vi "Calibrate Probe Tube.vi"(5 "Right":string="SN24", 7 "Left":string="SN31", 9 "Outputs":T14[](array[typedef])=[{"Name"="Right primary", "Device"="Dev1/ao0"}, {"Name"="Right secondary", "Device"="Dev1/ao1"}, {"Name"="Left primary", "Device"=""}, {"Name"="Left secondary", "Device"=""}, {"Name"="Shaker", "Device"=""}, {"Name"="Background", "Device"=""}], 11 "Inputs":T14[](array[typedef])=[{"Name"="Probe Mic Right", "Device"="Dev1/ai0"}, {"Name"="Probe Mic Left", "Device"=""}, {"Name"="Cal Mic", "Device"="Dev1/ai1"}, {"Name"="ABR", "Device"=""}, {"Name"="CAP Right", "Device"=""}, {"Name"="CAP Left", "Device"=""}, {"Name"="Accelerometer", "Device"=""}, {"Name"="Temperature", "Device"=""}, {"Name"="Heart rate", "Device"=""}]) -> ()   [LabVIEW 2020]
uses:
  <vilib>/printing/EasyPrintingControls.llb/layout_options.ctl
  <vilib>/printing/EasyPrintingControls.llb/orientation.ctl
  <vilib>/printing/EasyPrintingControls.llb/panel_scaling_for_page.ctl
  <vilib>/printing/EasyPrintingControls.llb/margins.ctl
  <vilib>/printing/EasyPrintingControls.llb/margin_values.ctl
  <vilib>/printing/EasyPrintingControls.llb/measurement_system.ctl
  <vilib>/printing/EasyPrintingControls.llb/printer_options.ctl
  <vilib>/printing/EasyPrintingControls.llb/printing_method.ctl
  <vilib>/printing/EasyPrintingControls.llb/color_or_monochrome.ctl
  <vilib>/printing/EasyPrintingControls.llb/page_header_options.ctl
  <vilib>/printing/EasyPrintingControls.llb/page_headers.ctl
  <vilib>/printing/EasyPrintingControls.llb/page_header_content_options.ctl
  epl-vi-lib/Utility VIs/Controls/KLegend/KLegend.xctl
  Common VIs/Typedefs/CAL-Endpoint.ctl
  Typedefs/PTC-Parameters.ctl
  Common VIs/Typedefs/CAL-Stimulus.ctl
  Typedefs/PTC-Queue Data.ctl
  Typedefs/PTC-Response.ctl
  epl-vi-lib/PXI DAQ VIs/AIDI/Typedefs/AIDI-Action.ctl
  <vilib>/printing/EasyPrintingControls.llb/contents.ctl
  7e04b9d2-1ebf-4042-b86f-09db3b0598e0.vi
  3dd90dd6-0296-4ee9-b2b6-3c947d5e5bcc.vi
  Common VIs/Typedefs/CAL-Globals.vi
  epl-vi-lib/Utility VIs/Math VIs/FFT x(t) to dB,Degrees (2D).vi
  epl-vi-lib/Utility VIs/Conversion VIs/Create Waveform Cluster (2D).vi
  epl-vi-lib/Utility VIs/File IO VIs/FileIO-Create Backup.vi
  epl-vi-lib/Utility VIs/File IO VIs/Append to Text File.vi
  <vilib>/printing/EasyPrinting.llb/Easy Print VI Panel or Documentation (refnum).vi
  <vilib>/Utility/NIReport.llb/NI_ReportGenerationCore.lvlib
panel:
  out "Acquired":i32=256
  in  "layout options":T1={"orientation (unchanged)"=0, "panel scaling for page (unchanged)"=0, "margins"={"override VI margins (false)"=FALSE, "margins (1.00)"={"top"=1.0, "left"=1.0, "right"=1.0, "bottom"=1.0}, "measurement system (default)"=0}, "printer options"={"destination printer name (current)"="", "printing method (unchanged)"=0, "color or monochrome (unchanged)"=0}, "page header options"={"page headers (unchanged)"=0, "page header content options"={"Include VI Name"=TRUE, "Include VI Path"=TRUE, "Include Last Modification Date"=TRUE, "Include Date Printed"=TRUE, "Include Page Number"=TRUE, "Include VI Icon"=TRUE}}} {"page header options"."page headers (unchanged)" items=["Unchanged", "Include page headers", "Do not include page headers"]; "printer options"."color or monochrome (unchanged)" items=["Unchanged", "Color/grayscale", "Monochrome"]; "printer options"."printing method (unchanged)" items=["Unchanged", "Standard", "PostScript", "Bitmap"]; "panel scaling for page (unchanged)" items=["Unchanged", "No Scaling", "Scale front panel to fit"]; "orientation (unchanged)" items=["Unchanged", "portrait", "landscape"]; "margins"."measurement system (default)" items=["Default", "US", "Metric"]; "margins"."margins (1.00)"."right" format="%.2f"; "margins"."margins (1.00)"."bottom" format="%.2f"; "margins"."margins (1.00)"."top" format="%.2f"; "margins"."margins (1.00)"."left" format="%.2f"}
  in  "Correction curve":path
  in  "Measure":bool
  out "(mV/Pa)":dbl=40.0 format="%#_4g"
  in  "Acoustic System ID":string="SN31"
  in  "Ear":enum16{"Right", "Left"}(ring)
  in  "Probe Mic Gain (dB)":dbl
  in  "Cal Mic Gain (dB)":dbl=40.0
  in  "Stimulus":T13={"Freq Step (Hz)"=50.0, "Stimulus"=enum."Chirp", "Attenuation (dB)"=30.0, "Sample Rate (Hz)"=100000.0}
  in  "Averages":i32=256
  in  "Cal Mic Sens":dbl=-146.12351367888365 caption="(dB V/SPL)" format="%.2f"
  in  "RETURN":bool
  in  "START":bool
  in  "STOP":bool
  out "result":cluster{"Path":path, "error":errorcluster}
  in  "Data tabs":enum32{"Raw", "Calibration"}(tab)
  out "Mic mag":cluster{"offset":dbl, "dx":dbl, "Y":dbl[][]}(graph)
  out "Mic signals":cluster{"offset":dbl, "dx":dbl, "Y":dbl[][]}(graph)
  in  "KLegend":i32(xcontrol)
  out "PT mag":cluster{"PTC Mag":dbl[], "PTC Phase":dbl[]}[](graph)
  in  "Open Button":bool
  in  "Clear Button":bool
  in  "Smooth Button":bool
  in  "Validate Button":bool
  out "Path":path
  out "PT phase":cluster{"PTC Mag":dbl[], "PTC Phase":dbl[]}[](graph)
  # "Calibrated Mic Sensitivity"
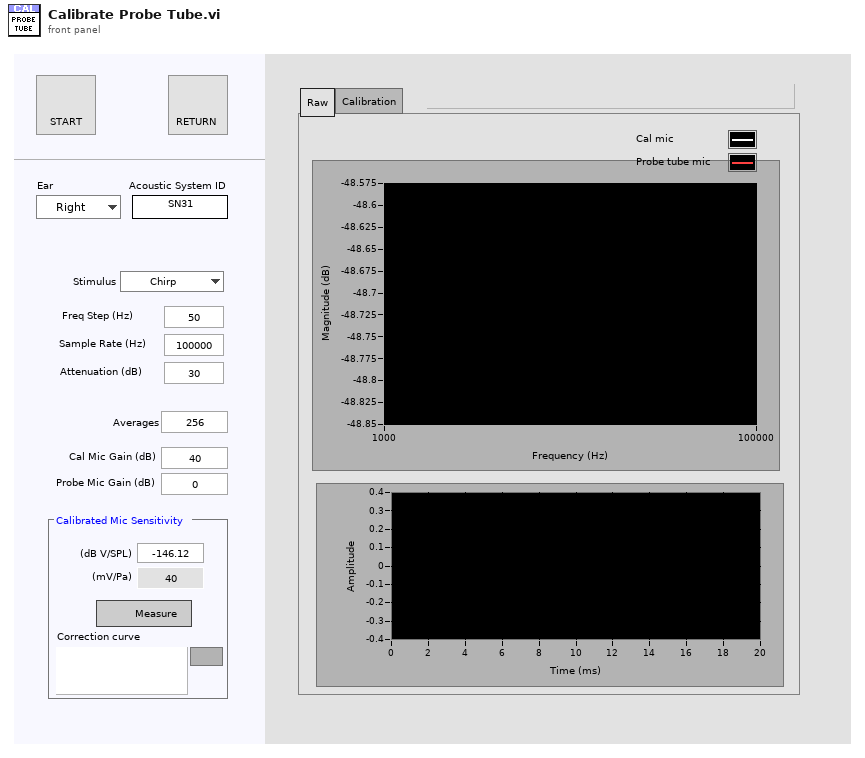
[diagram p1: front panel]
types:
  T1 = typedef "NI_ReportGenerationCore.lvlib/layout_options.ctl" = cluster{"orientation (unchanged)":T2, "panel scaling for page (unchanged)":T3, "margins":T4, "printer options":T7, "page header options":T10}
  T2 = typedef "NI_ReportGenerationCore.lvlib/orientation.ctl" = u16
  T3 = typedef "NI_ReportGenerationCore.lvlib/panel_scaling_for_page.ctl" = u16
  T4 = typedef "NI_ReportGenerationCore.lvlib/margins.ctl" = cluster{"override VI margins (false)":bool, "margins (1.00)":T5, "measurement system (default)":T6}
  T5 = typedef "NI_ReportGenerationCore.lvlib/margin_values.ctl" = cluster{"top":dbl, "left":dbl, "right":dbl, "bottom":dbl}
  T6 = typedef "NI_ReportGenerationCore.lvlib/measurement_system.ctl" = u16
  T7 = typedef "NI_ReportGenerationCore.lvlib/printer_options.ctl" = cluster{"destination printer name (current)":string, "printing method (unchanged)":T8, "color or monochrome (unchanged)":T9}
  T8 = typedef "NI_ReportGenerationCore.lvlib/printing_method.ctl" = u16
  T9 = typedef "NI_ReportGenerationCore.lvlib/color_or_monochrome.ctl" = u16
  T10 = typedef "NI_ReportGenerationCore.lvlib/page_header_options.ctl" = cluster{"page headers (unchanged)":T11, "page header content options":T12}
  T11 = typedef "NI_ReportGenerationCore.lvlib/page_headers.ctl" = u16
  T12 = typedef "NI_ReportGenerationCore.lvlib/page_header_content_options.ctl" = cluster{"Include VI Name":bool, "Include VI Path":bool, "Include Last Modification Date":bool, "Include Date Printed":bool, "Include Page Number":bool, "Include VI Icon":bool}
  T13 = cluster{"Freq Step (Hz)":dbl, "Stimulus":enum16{"Chirp"}, "Attenuation (dB)":dbl, "Sample Rate (Hz)":dbl}
  T14 = typedef "CAL-Endpoint.ctl" = cluster{"Name":string, "Device":string}
  T15 = typedef "PTC-Queue Data.ctl" = cluster{"action":string, "Speaker":string, "Probe mic":string, "Cal mic":string, "ID":string, "Stimulus":T16, "Response":T17, "Mic corr":path}
  T16 = typedef "CAL-Stimulus.ctl" = cluster{"Type":string, "Freq step (Hz)":dbl, "Sampling rate (Hz)":dbl, "Attenuation (dB)":dbl}
  T17 = typedef "PTC-Response.ctl" = cluster{"Cal mic gain":dbl, "Probe mic gain":dbl, "Cal mic sens":dbl, "Averages":i32}
  T18 = cluster{"Right":string, "Left":string, "Outputs":T14[], "Inputs":T14[]}
  T19 = typedef "PTC-Parameters.ctl" = cluster{"Ear":enum16{"Right", "Left"}, "Stimulus":T16, "Averages":i32, "Cal Mic Gain":dbl, "Probe Mic Gain":dbl, "Cal Mic Sens":dbl, "Correction":path}
  T20 = typedef "AIDI-Action.ctl" = enum16{"Configure", "Initialize", "Start", "Read", "Clean up", "Init & Start", "Config & Test", "Position", "Skip"}
  T21 = typedef "CAL-Data.ctl" = cluster{"Freq (Hz)":dbl[], "Magnitude (dB SPL/V)":dbl[], "Phase (degrees)":dbl[]}
  T22 = cluster{"Path (out)":path, "error out":errorcluster}
  T23 = typedef "NI_ReportGenerationCore.lvlib/contents.ctl" = u16
  T24 = typedef "TDT-Device Config.ctl" = cluster{"Output":T25, "Input":T27}
  T25 = typedef "TDT-Output source.ctl" = cluster{"Device":T26, "Num":i32}
  T26 = typedef "TDT-Device ID.ctl" = enum16{"None", "PA5", "RP2", "RL2", "RA16", "RV8", "RX5", "RX6", "RX7", "RX8", "RZ2", "RZ5", "RZ6"}
  T27 = typedef "TDT-Input source.ctl" = enum16{"Front Panel", "RA4LI", "RA16LI"}
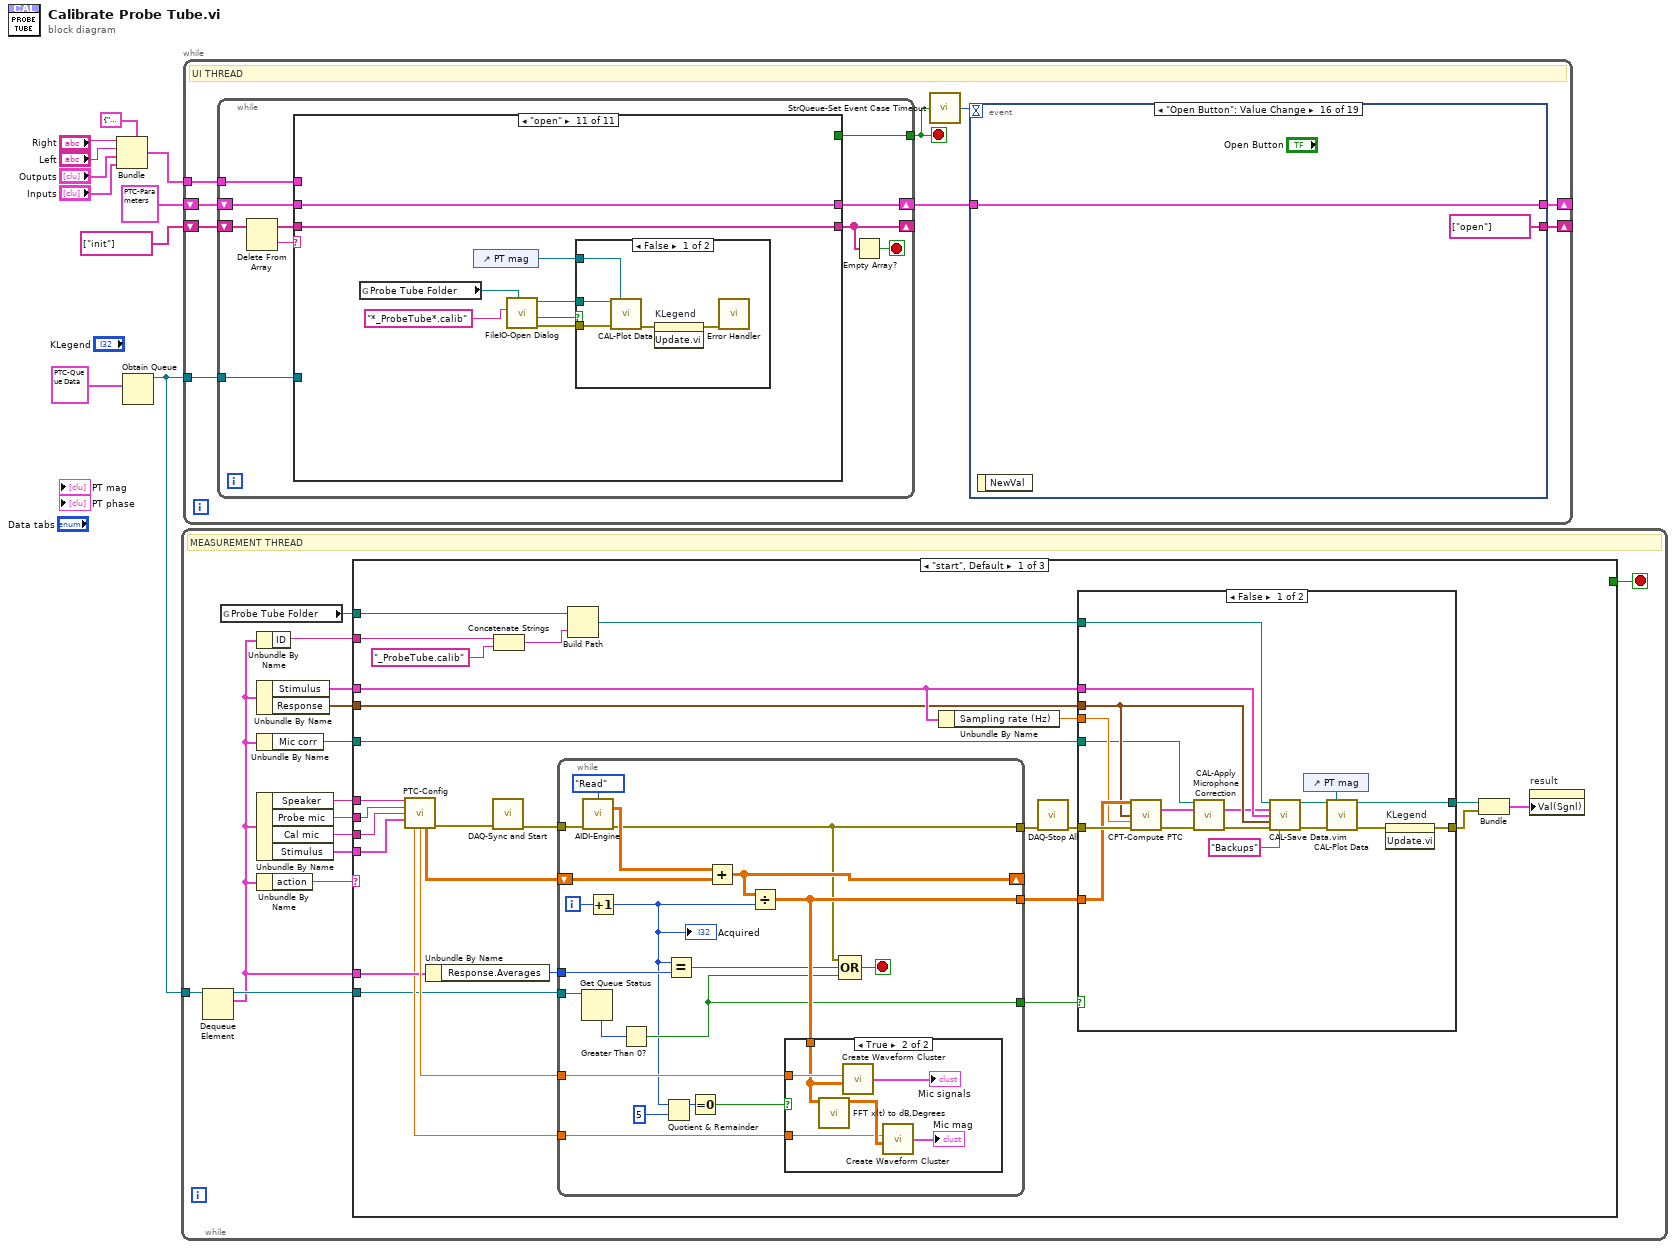
[diagram p0: block diagram]
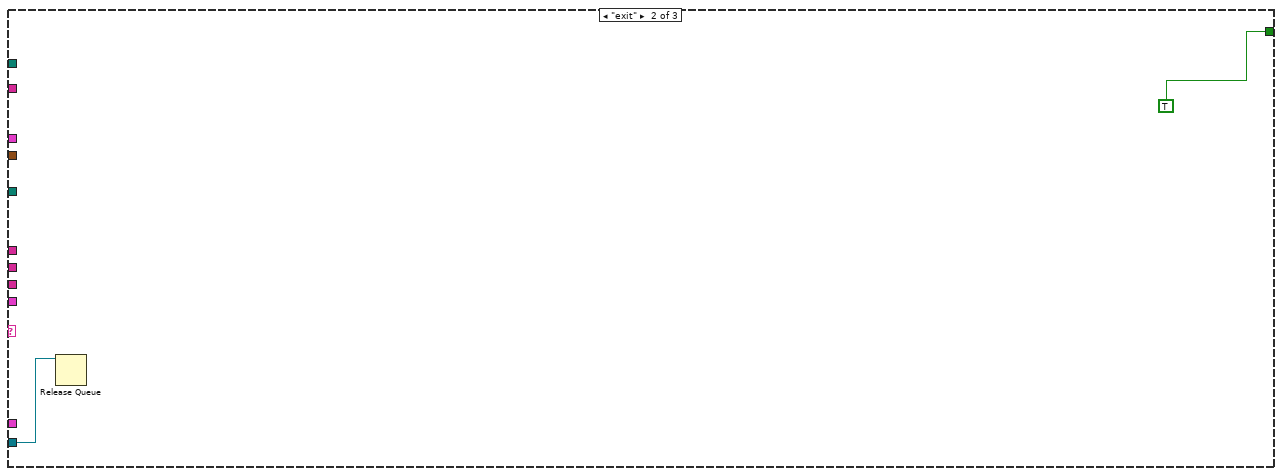
[diagram p4: hidden frame]
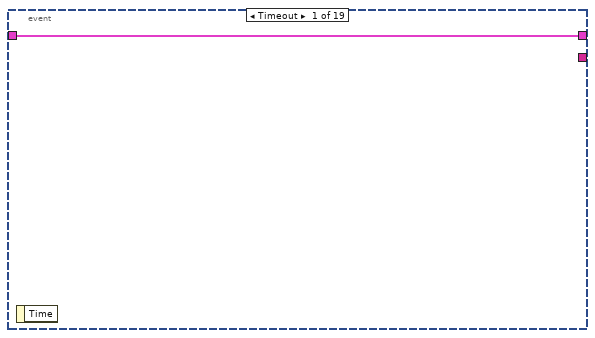
[diagram p6: hidden frame]
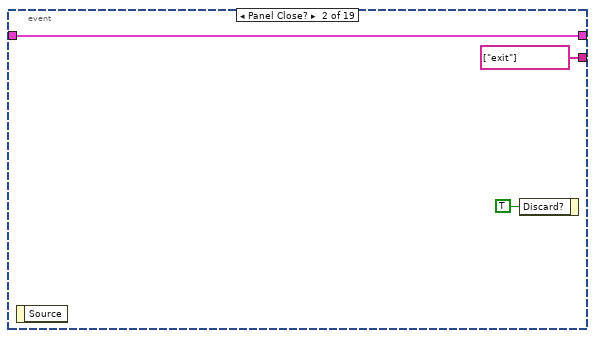
[diagram p7: hidden frame]
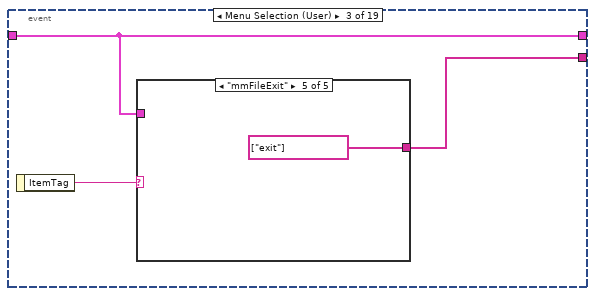
[diagram p8: hidden frame]
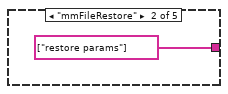
[diagram p10: hidden frame]
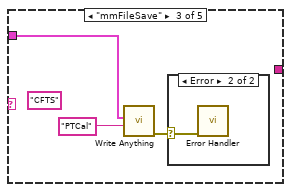
[diagram p11: hidden frame]
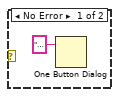
[diagram p12: hidden frame]
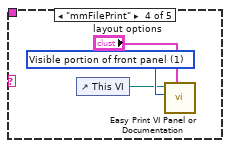
[diagram p13: hidden frame]
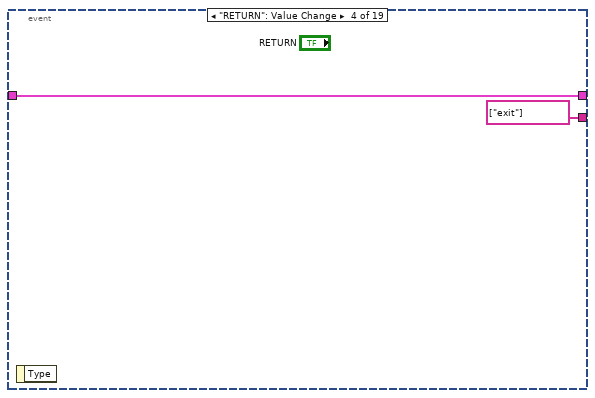
[diagram p14: hidden frame]
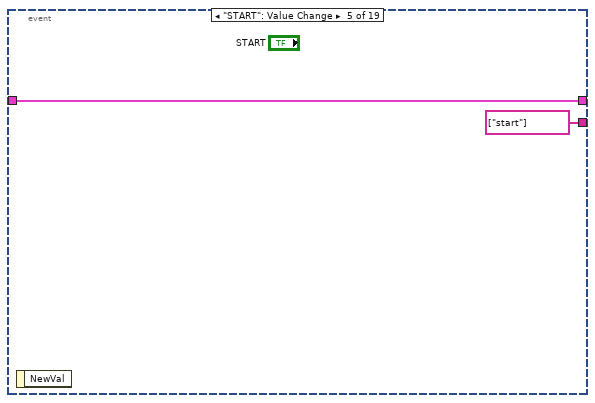
[diagram p15: hidden frame]
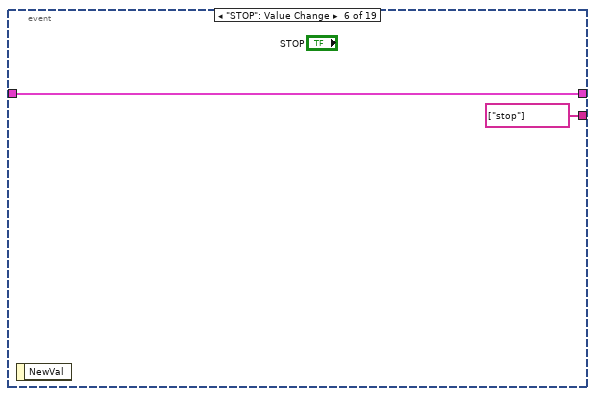
[diagram p16: hidden frame]
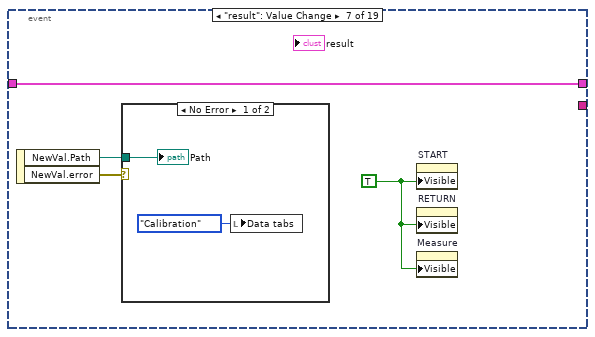
[diagram p17: hidden frame]
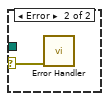
[diagram p18: hidden frame]
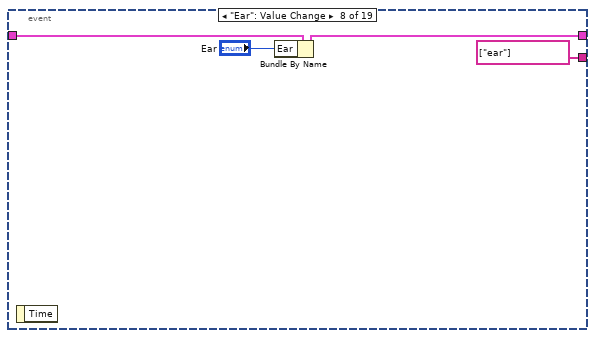
[diagram p19: hidden frame]
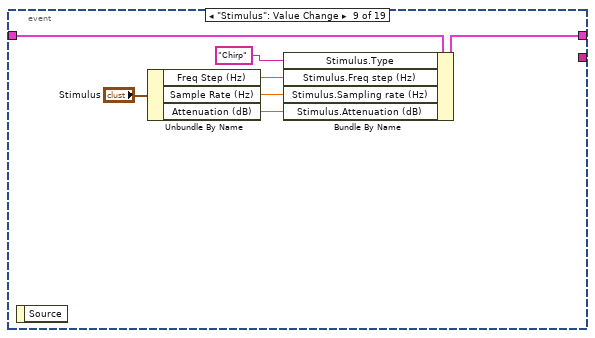
[diagram p20: hidden frame]
diagram:
  n1 = Bundle(cluster=T18 {"Right"="", "Left"="", "Outputs"=[], "Inputs"=[]}, "Right"="Right", "Left"="Left", "Outputs"="Outputs", "Inputs"="Inputs") -> (w2:T18)
  n2 = Obtain Queue(element data type=T15 {"action"="", "Speaker"="", "Probe mic"="", "Cal mic"="", "ID"="", "Stimulus"={"Type"="", "Freq step (Hz)"=0.0, "Sampling rate (Hz)"=0.0, "Attenuation (dB)"=0.0}, "Response"={"Cal mic gain"=0.0, "Probe mic gain"=0.0, "Cal mic sens"=0.0, "Averages"=0}, "Mic corr"=path ""} ("data")) -> (queue out=w10:refnum<queue>)  [unwired: 4 in, 2 out]
  n3 = while {
    tunnel: w10 -> [w24]
    stop <- w21 stop-if-true
    # "MEASUREMENT THREAD"
    n4 = Dequeue Element(queue=w24) -> (queue out=w22:refnum<queue>, element=w12:T15)  [unwired: 2 in, 2 out]
    n5 = global read "CAL-Globals.vi" "Probe Tube Folder"() -> (w15:path)
    n6 = Unbundle By Name(w12) -> ("ID"=w16:string)
    n7 = Unbundle By Name(w12) -> ("Stimulus"=w13:T16, "Response"=w14:T17)
    n8 = Unbundle By Name(w12) -> ("Mic corr"=w11:path)
    n9 = Unbundle By Name(w12) -> ("Speaker"=w20:string, "Probe mic"=w19:string, "Cal mic"=w18:string, "Stimulus"=w17:T16)
    n10 = Unbundle By Name(w12) -> ("action"=w23:string)
    n11 = case shown="\"start\", Default" w23 {
      tunnel: w22 -> [w40 w99 _]
      tunnel: [_ TRUE _] -> w21
      tunnel: w20 -> [w52 _ _]
      tunnel: w19 -> [w51 _ _]
      tunnel: w18 -> [w50 _ _]
      tunnel: w17 -> [w49 _ _]
      tunnel: w12 -> [w42 _ _]
      tunnel: w16 -> [w37 _ _]
      tunnel: w15 -> [w36 _ _]
      tunnel: w14 -> [w31 _ _]
      tunnel: w13 -> [w32 _ _]
      tunnel: w11 -> [w25 _ _]
      frame "start", Default {
        n12 = call "PTC-Config.vi"("Speaker"=w52, "Probe mic"=w51, "Cal mic"=w50, "Stimulus"=w49) -> ("df (Hz)"=w41:dbl, "dt (ms)"=w43:dbl, "Mic Avg"=w44:dbl[][], "error out"=w45:errorcluster)  [unwired: 8 in]
        n13 = Unbundle By Name(w42) -> ("Response.Averages"=w47:i32)
        n14 = call "DAQ-Sync and Start.vi"("error in (no error)"=w45) -> ("error out"=w48:errorcluster)  [unwired: 14 in]
        n15 = Concatenate Strings(w37, "_ProbeTube.calib" ("string")) -> (w35:string)
        n16 = while {
          tunnel: [w72] -> w46
          shift-right: [w89] -> _
          shift-left: w44 -> [w90]
          tunnel: [w84] -> w38
          tunnel: w41 -> [w86]
          tunnel: w43 -> [w85]
          tunnel: w47 -> [w83]
          tunnel: w48 -> [w81]
          tunnel: w40 -> [w79]
          tunnel: [w75] -> w29
          i -> [w91]
          stop <- w87 stop-if-true
          n17 = Get Queue Status(queue=w79) -> (# elements in queue=w78:i32)  [unwired: 2 in, 7 out]
          n18 = call "AIDI-Engine.vi"("Action"=AIDI-Action."Read", "error in (no error)"=w81) -> ("AI"=w73:dbl[][], "error out"=w72:errorcluster)  [unwired: 8 in, 4 out]
          n19 = Increment(x=w91) -> (x+1=w74:i32)
          "Acquired" <- w74
          n20 = Greater Than 0?(x=w78) -> (x > 0?=w75:bool)
          n21 = Quotient & Remainder(x=w74, y=5) -> (x-y*floor(x/y)=w88:i32)  [unwired: 1 out]
          n22 = Equal?(x=w74, y=w83) -> (x = y?=w76:bool)
          n23 = Equal To 0?(x=w88) -> (x = 0?=w77:bool)
          n24 = Add(x=w73, y=w90) -> (x+y=w89:dbl[][])
          n25 = Divide(x=w89, y=w74) -> (x/y=w84:dbl[][])
          n26 = case shown="True" w77 {
            tunnel: w86 -> [_ w93]
            tunnel: w85 -> [_ w95]
            tunnel: w84 -> [_ w92]
            frame False {
            }
            frame True {
              n27 = call-poly "FFT x(t) to dB,Degrees.vi"("X(t)"=w92) -> ("+Freq. Mag of FFT (dB rms)"=w96:dbl[][])  [unwired: 8 in, 2 out]
              n28 = call-poly "Create Waveform Cluster.vi"("dx"=w95, "Array"=w92) -> ("waveform cluster"=→"Mic signals":cluster{"offset":dbl, "dx":dbl, "Y":dbl[][]})  [unwired: 3 in]
              n29 = call-poly "Create Waveform Cluster.vi"("dx"=w93, "Array"=w96) -> ("waveform cluster"=→"Mic mag":cluster{"offset":dbl, "dx":dbl, "Y":dbl[][]})  [unwired: 3 in]
            }
          }
          n30 = Compound Arithmetic op=OR(w72, w76, w75) -> (w87:bool)
        }
        n31 = Build Path(base path=w36, name or relative path=w35) -> (appended path=w30:path)
        n32 = Unbundle By Name(w32) -> ("Sampling rate (Hz)"=w33:dbl)
        n33 = call "DAQ-Stop All.vi"("error in (no error)"=w46) -> ("error out"=w39:errorcluster)  [unwired: 14 in]
        n34 = case shown="False" w29 {
          tunnel: w39 -> [w70 w71]
          tunnel: w38 -> [w69 _]
          tunnel: w33 -> [w68 _]
          tunnel: w32 -> [w67 _]
          tunnel: w31 -> [w66 _]
          tunnel: w30 -> [w65 _]
          tunnel: [w60 w71] -> w27
          tunnel: [w59 _] -> w28
          tunnel: w25 -> [w54 _]
          frame False {
            n35 = call "CPT-Compute PTC.vi"(0:"Response"=w69, 7:"Response"=w66, "Fs (Hz)"=w68, "error in (no error)"=w70) -> ("data"=w57:T21, "error out"=w58:errorcluster)  [unwired: 10 in]
            n36 = call "CAL-Apply Microphone Correction.vi"("Correction curve"=w54, "data"=w57, "error in (no error)"=w58) -> ("corrected data"=w56:T21, "error out"=w55:errorcluster)  [unwired: 11 in]
            n37 = call "CAL-Save Data.vim"("path"=w65, "Data"=w56, "Stimulus"=w67, "Response"=w66, "error in (no error)"=w55, "Backup folder"="Backups") -> ("new file path"=w64:path, "error out"=w63:errorcluster)  [unwired: 8 in]
            n38 = control-ref of="PT mag"() -> (w62:refnum<vi>)
            n39 = call "CAL-Plot Data.vi"("Path"=w64, "Mag graph"=w62, "error in (no error)"=w63) -> ("Path (out)"=w59:path, "error out"=w61:errorcluster)  [unwired: 11 in]
            n40 = invoke on="KLegend" class="KLegend (strict)" method="Update.vi"(error in=w61) -> (error out=w60:errorcluster)  [unwired: 2 in, 2 out]
          }
          frame True {
          }
        }
        n41 = Bundle("Path (out)"=w28, "error out"=w27) -> (w26:T22)  [unwired: 1 in]
        n42 = property on="result" class="Clust (strict)"("Val(Sgnl)"=w26) -> ()  [unwired: 2 in, 2 out]
      }
      frame "exit" {
        n43 = Release Queue(queue=w99) -> ()  [unwired: 2 in, 3 out]
      }
      frame "stop" {
      }
    }
  }
  n44 = while {
    tunnel: w10 -> [w101]
    shift-right: [w102] -> _
    shift-left: T19 {"Ear"=enum."Right", "Stimulus"={"Type"="", "Freq step (Hz)"=50.0, "Sampling rate (Hz)"=50000.0, "Attenuation (dB)"=20.0}, "Averages"=512, "Cal Mic Gain"=40.0, "Probe Mic Gain"=40.0, "Cal Mic Sens"=-156.0, "Correction"=path ""} ("Params") -> [w108]
    shift-right: [w107] -> _
    shift-left: string[] ["init"] -> [w106]
    tunnel: w2 -> [w100]
    stop <- w104 stop-if-true
    # "UI THREAD"
    n45 = while {
      shift-right: [w211] -> _
      shift-left: w106 -> [w214]
      tunnel: w101 -> [w209]
      tunnel: [w208] -> w104
      shift-right: [w206] -> w103
      shift-left: w108 -> [w207]
      tunnel: w100 -> [w205]
      stop <- w210 stop-if-true
      n46 = Delete From Array(array=w214) -> (deleted portion=w212:string, array with subset deleted=w213:string[])  [unwired: 2 in]
      n47 = case shown="\"open\"" w212 {
        tunnel: w213 -> [w216 w223 w229 _ w240 w256 w265 w273 w278 w286 w299]
        tunnel: [w216 w223 w229 string[] ["restore defaults", "clear"] w239 w248 w265 w273 w278 w286 w299] -> w211
        tunnel: w209 -> [_ w220 w227 _ _ _ _ _ _ w282 _]
        tunnel: [_ TRUE _ _ _ _ _ _ _ _ _] -> w208
        tunnel: w207 -> [w215 w221 w228 w235 _ w255 w264 w272 w276 w284 w298]
        tunnel: [w215 w221 w228 w235 w237 w255 w264 w272 w276 w284 w298] -> w206
        tunnel: w205 -> [_ _ _ _ _ _ w259 _ _ w283 _]
        frame "", Default {
        }
        frame "exit" {
          n48 = Bundle By Name(cluster=T15 {"action"="", "Speaker"="", "Probe mic"="", "Cal mic"="", "ID"="", "Stimulus"={"Type"="", "Freq step (Hz)"=0.0, "Sampling rate (Hz)"=0.0, "Attenuation (dB)"=0.0}, "Response"={"Cal mic gain"=0.0, "Probe mic gain"=0.0, "Cal mic sens"=0.0, "Averages"=0}, "Mic corr"=path ""} ("data"), "action"="exit") -> (w217:T15)
          n49 = Enqueue Element(queue=w220, element=w217) -> ()  [unwired: 2 in, 3 out]
        }
        frame "stop" {
          n50 = Bundle By Name(cluster=T15 {"action"="", "Speaker"="", "Probe mic"="", "Cal mic"="", "ID"="", "Stimulus"={"Type"="", "Freq step (Hz)"=0.0, "Sampling rate (Hz)"=0.0, "Attenuation (dB)"=0.0}, "Response"={"Cal mic gain"=0.0, "Probe mic gain"=0.0, "Cal mic sens"=0.0, "Averages"=0}, "Mic corr"=path ""} ("data"), "action"="stop") -> (w224:T15)
          n51 = Enqueue Element(queue=w227, element=w224) -> ()  [unwired: 2 in, 3 out]
        }
        frame "init" {
          w233 = TRUE ("Visible")
          n52 = global read "CAL-Globals.vi" "Probe Tube Folder"() -> (w232:path)
          n53 = control-ref of="PT mag"() -> (w230:refnum<vi>)
          n54 = call "FileIO-File or Folder Exists.vi"("path"=w232) -> ("Exists?"=w231:bool)  [unwired: 7 in, 3 out]
          n55 = property on="KLegend" class="KLegend (strict)"("Plot refnum"=w230) -> ()  [unwired: 2 in, 2 out]
          n56 = case shown="False" w231 {
            tunnel: w232 -> [w236 _]
            frame False {
              n57 = Create Folder(path (use dialog)=w236) -> ()  [unwired: 2 in, 3 out]
            }
            frame True {
            }
          }
          n58 = property on="RETURN" class="Bool"("Visible"=w233) -> ()  [unwired: 2 in, 2 out]
          n59 = property on="START" class="Bool"("Visible"=w233) -> ()  [unwired: 2 in, 2 out]
        }
        frame "restore defaults" {
          n60 = call "PTC-Restore Defaults.vi"() -> ("Params"=w237:T19)  [unwired: 14 in, 1 out]
          n61 = Build Array (concatenate)(w240, "show") -> (w239:string[])
        }
        frame "show" {
          n62 = Unbundle By Name(w255) -> ("Ear"=w254:enum16{"Right", "Left"}, "Averages"=w253:i32, "Cal Mic Gain"=w252:dbl, "Probe Mic Gain"=w251:dbl, "Cal Mic Sens"=w250:dbl, "Correction"=w249:path, "Stimulus.Freq step (Hz)"=w244:dbl, "Stimulus.Sampling rate (Hz)"=w243:dbl, "Stimulus.Attenuation (dB)"=w242:dbl)
          n63 = local write "Ear"(w254) -> ()
          n64 = local write "Averages"(w253) -> ()
          n65 = local write "Cal Mic Gain (dB)"(w252) -> ()
          n66 = local write "Probe Mic Gain (dB)"(w251) -> ()
          n67 = local write "Cal Mic Sens"(w250) -> ()
          n68 = local write "Correction curve"(w249) -> ()
          n69 = local read "Stimulus"() -> (w245:T13)
          n70 = Bundle By Name(cluster=w245, "Freq Step (Hz)"=w244, "Sample Rate (Hz)"=w243, "Attenuation (dB)"=w242) -> (w241:T13)
          n71 = local write "Stimulus"(w241) -> ()
          n72 = Build Array (concatenate)(w256, "ear", "cal mic sens") -> (w248:string[])
        }
        frame "ear" {
          n73 = Unbundle By Name(w259) -> ("Right"=w258:string, "Left"=w257:string)
          n74 = Unbundle By Name(w264) -> ("Ear"=w262:enum16{"Right", "Left"})
          n75 = Equal?(x=enum16{"Right", "Left"}."Right", y=w262) -> (x = y?=w263:bool)
          n76 = Select(t=w258, s=w263, f=w257) -> (s? t:f=w260:string)
          n77 = local write "Acoustic System ID"(w260) -> ()
        }
        frame "cal mic sens" {
          n78 = Unbundle By Name(w272) -> ("Cal Mic Sens"=w266:dbl)
          n79 = call "Math-dB To Linear.vim"("dB"=w266) -> ("linear"=w267:dbl)
          n80 = Divide(x=w267, y=2e-05) -> (x/y=w269:dbl)
          n81 = Multiply(x=w269, y=1000.0) -> (x*y=→"(mV/Pa)":dbl)
        }
        frame "clear" {
          w274 = cluster{"offset":dbl, "dx":dbl, "Y":dbl[][]} {"offset"=0.0, "dx"=0.005, "Y"=[]} ("Mic signals")
          w275 = cluster{"PTC Mag":dbl[], "PTC Phase":dbl[]}[] [] ("PT mag graph")
          n82 = property on="PT mag" class="XYGraph (strict)"("Value"=w275, "Legend Visible"=FALSE ("Legend:Visible")) -> ()  [unwired: 2 in, 2 out]
          n83 = property on="PT phase" class="XYGraph (strict)"("Value"=w275) -> ()  [unwired: 2 in, 2 out]
          n84 = local write "Mic signals"(w274) -> ()
          n85 = local write "Mic mag"(w274) -> ()
        }
        frame "start" {
          n86 = local write "Data tabs"(enum32{"Raw", "Calibration"}."Raw" ("Data tabs")) -> ()
          n87 = call "PTC-Create Queue Data.vi"("state"=w283, "Params"=w284, "Acoustic System ID"="Acoustic System ID") -> ("data"=w281:T15, "error out"=w279:errorcluster)  [unwired: 11 in]
          n88 = case shown="No Error" w279 {
            selector: w279 -> [_ w291]
            tunnel: w282 -> [w290 _]
            tunnel: w281 -> [w289 _]
            frame No Error {
              w288 = FALSE
              n89 = Enqueue Element(queue=w290, element=w289) -> ()  [unwired: 2 in, 3 out]
              n90 = local write "Path"(path "" ("Path")) -> ()
              n91 = property on="RETURN" class="Bool"("Visible"=w288) -> ()  [unwired: 2 in, 2 out]
              n92 = property on="START" class="Bool"("Visible"=w288) -> ()  [unwired: 2 in, 2 out]
              n93 = property on="Measure" class="Bool"("Visible"=w288) -> ()  [unwired: 2 in, 2 out]
            }
            frame Error {
              n94 = call "Error Handler.vi"("error in (no error)"=w291) -> ()  [unwired: 13 in, 2 out]
            }
          }
        }
        frame "open" {
          n95 = global read "CAL-Globals.vi" "Probe Tube Folder"() -> (w296:path)
          n96 = control-ref of="PT mag"() -> (w297:refnum<vi>)
          n97 = call "FileIO-Open Dialog.vi"("Default Folder"=w296, "pattern (all files)"="*_ProbeTube*.calib") -> ("error out"=w292:errorcluster, "cancelled"=w294:bool, "selected path"=w293:path)  [unwired: 7 in]
          n98 = case shown="False" w294 {
            tunnel: w297 -> [w302 _]
            tunnel: w293 -> [w304 _]
            tunnel: w292 -> [w303 _]
            frame False {
              n99 = call "CAL-Plot Data.vi"("Path"=w304, "Mag graph"=w302, "error in (no error)"=w303) -> ("error out"=w301:errorcluster)  [unwired: 11 in, 1 out]
              n100 = invoke on="KLegend" class="KLegend (strict)" method="Update.vi"(error in=w301) -> (error out=w300:errorcluster)  [unwired: 2 in, 2 out]
              n101 = call "Error Handler.vi"("error in (no error)"=w300) -> ()  [unwired: 13 in, 2 out]
            }
            frame True {
            }
          }
        }
      }
      n102 = Empty Array?(array=w211) -> (empty?=w210:bool)
    }
    n103 = call "StrQueue-Set Event Case Timeout.vi"("Quit"=w104) -> ("timeout"=w105:i32)  [unwired: 14 in]
    n104 = event shown="[15] \"Open Button\": Value Change" {
      selector: _ -> [_ _ _ _ _ _ _ _ _ _ _ _ _ _ _ _ _ _ _]
      dyn-events: _ -> [_ _ _ _ _ _ _ _ _ _ _ _ _ _ _ _ _ _ _]
      timeout: w105 -> [_ _ _ _ _ _ _ _ _ _ _ _ _ _ _ _ _ _ _]
      tunnel: [_ string[] ["exit"] w114 string[] ["exit"] string[] ["start"] string[] ["stop"] _ string[] ["ear"] _ _ string[] ["cal mic sens"] _ _ _ string[] ["cal mic sens"] string[] ["open"] string[] ["clear"] _ _] -> w107
      tunnel: [w109 w110 w113 w126 w129 w131 w133 w140 w148 w151 w155 w158 w161 w164 w168 w177 w178 w180 w192] -> w102
      tunnel: w103 -> [w109 w110 w113 w126 w129 w131 w133 w142 w149 w152 w156 w159 w162 w165 w167 w177 w178 w180 w192]
      event Timeout {
        n105 = event-data() -> ()  [unwired: 1 in, 1 out]
      }
      event Panel Close? {
        n106 = event-data() -> ()  [unwired: 1 in, 1 out]
        n107 = event-data("Discard?"=TRUE) -> ()  [unwired: 1 in, 1 out]
      }
      event Menu Selection (User) {
        n108 = event-data() -> ("ItemTag"=w115:string)  [unwired: 1 in]
        n109 = case shown="\"mmFileExit\"" w115 {
          tunnel: w113 -> [_ _ w118 _ _]
          tunnel: [_ string[] ["restore params"] _ _ string[] ["exit"]] -> w114
          frame "", Default {
          }
          frame "mmFileRestore" {
          }
          frame "mmFileSave" {
            (unwired) "CFTS" ("AppName")
            n110 = call "Write Anything.vi"("Section Name (Name of \"Anything\")"="PTCal" ("Section Name (Name of \"Type of Anything\")"), "Anything"=w118) -> ("Error Out"=w117:errorcluster)  [unwired: 8 in, 1 out]
            n111 = case shown="Error" w117 {
              selector: w117 -> [_ w121]
              frame No Error {
                n112 = One Button Dialog(message="Defaults saved.") -> ()  [unwired: 1 in, 1 out]
              }
              frame Error {
                n113 = call "Error Handler.vi"("error in (no error)"=w121) -> ()  [unwired: 13 in, 2 out]
              }
            }
          }
          frame "mmFilePrint" {
            w124 = T23 1 items=["Complete front panel", "Visible portion of front panel", "Icon, description, panel and diagram", "Documentation: Using the panel", "Documentation: Using as a subVI", "Documentation: Complete", "Documentation: Custom"] ("contents (complete front panel)")
            n114 = control-ref of="This VI"() -> (w122:refnum<vi>)
            n115 = call-poly <vilib>:"Easy Print VI Panel or Documentation.vi"("layout options"="layout options", "contents (complete front panel)"=w124, "VI reference"=w122) -> ()  [unwired: 7 in, 2 out]
          }
          frame "mmFileExit" {
          }
        }
      }
      event "RETURN": Value Change {
        n116 = event-data() -> ()  [unwired: 1 in, 1 out]
      }
      event "START": Value Change {
        n117 = event-data() -> ()  [unwired: 1 in, 1 out]
      }
      event "STOP": Value Change {
        n118 = event-data() -> ()  [unwired: 1 in, 1 out]
      }
      event "result": Value Change {
        w134 = TRUE
        n119 = event-data() -> ("NewVal.Path"=w132:path, "NewVal.error"=w135:errorcluster)  [unwired: 1 in]
        n120 = case shown="No Error" w135 {
          selector: w135 -> [_ w138]
          tunnel: w132 -> [w136 _]
          frame No Error {
            n121 = local write "Data tabs"(enum32{"Raw", "Calibration"}."Calibration" ("Data tabs")) -> ()
            "Path" <- w136
          }
          frame Error {
            n122 = call "Error Handler.vi"("error in (no error)"=w138) -> ()  [unwired: 13 in, 2 out]
          }
        }
        n123 = property on="START" class="Bool"("Visible"=w134) -> ()  [unwired: 2 in, 2 out]
        n124 = property on="RETURN" class="Bool"("Visible"=w134) -> ()  [unwired: 2 in, 2 out]
        n125 = property on="Measure" class="Bool"("Visible"=w134) -> ()  [unwired: 2 in, 2 out]
      }
      event "Ear": Value Change {
        n126 = event-data() -> ()  [unwired: 1 in, 1 out]
        n127 = Bundle By Name(cluster=w142, "Ear"="Ear") -> (w140:T19)
      }
      event "Stimulus": Value Change {
        n128 = event-data() -> ()  [unwired: 1 in, 1 out]
        n129 = Unbundle By Name("Stimulus") -> ("Freq Step (Hz)"=w146:dbl, "Sample Rate (Hz)"=w145:dbl, "Attenuation (dB)"=w144:dbl)
        n130 = Bundle By Name(cluster=w149, "Stimulus.Type"="Chirp", "Stimulus.Freq step (Hz)"=w146, "Stimulus.Sampling rate (Hz)"=w145, "Stimulus.Attenuation (dB)"=w144) -> (w148:T19)
      }
      event "Averages": Value Change {
        n131 = event-data() -> ()  [unwired: 1 in, 1 out]
        n132 = Bundle By Name(cluster=w152, "Averages"="Averages") -> (w151:T19)
      }
      event "Cal Mic Sens": Value Change {
        n133 = event-data() -> ("NewVal"=w153:dbl)  [unwired: 1 in]
        n134 = Bundle By Name(cluster=w156, "Cal Mic Sens"=w153) -> (w155:T19)
      }
      event "Cal Mic Gain (dB)": Value Change {
        n135 = event-data() -> ("NewVal"=w157:dbl)  [unwired: 1 in]
        n136 = Bundle By Name(cluster=w159, "Cal Mic Gain"=w157) -> (w158:T19)
      }
      event "Probe Mic Gain (dB)": Value Change {
        n137 = event-data() -> ("NewVal"=w160:dbl)  [unwired: 1 in]
        n138 = Bundle By Name(cluster=w162, "Probe Mic Gain"=w160) -> (w161:T19)
      }
      event "Correction curve": Value Change {
        n139 = event-data() -> ()  [unwired: 1 in, 1 out]
        n140 = Bundle By Name(cluster=w165, "Correction"="Correction curve") -> (w164:T19)
      }
      event "Measure": Value Change {
        n141 = event-data() -> ()  [unwired: 1 in, 1 out]
        n142 = disable-structure shown="Disabled" {
          disable-tunnel: [w175 _] -> w168
          disable-tunnel: w167 -> [w174 _]
          frame Disabled {
            n143 = Unbundle By Name(w174) -> ("Cal Mic Sens"=w172:dbl)
            n144 = call "Cxns-Get Connections File Path.vi"() -> ("Path Out"=w171:path)  [unwired: 1 in]
            n145 = call "Equip-Get Device (TDT).vi"("Path In"=w171) -> ("TDT-Device Config"=w170:T24)  [unwired: 12 in, 2 out]
            n146 = call "Cal Mic Sensitivity (TDT).vi"("Device Config"=w170, "Mic Sens (dB V/SPL) in"=w172) -> ("Mic Sens (dB V/SPL)"=w169:dbl, "User ID"=w173:string)  [unwired: 8 in]
            n147 = Bundle By Name(cluster=w174, "Cal Mic Sens"=w169) -> (w175:T19)
            n148 = local write "Cal Mic Sens"(w169) -> ()
          }
          frame Enabled {
          }
        }
      }
      event "Open Button": Value Change {
        n149 = event-data() -> ()  [unwired: 1 in, 1 out]
      }
      event "Clear Button": Value Change {
        n150 = event-data() -> ()  [unwired: 1 in, 1 out]
      }
      event "Smooth Button": Value Change {
        n151 = event-data() -> ()  [unwired: 1 in, 1 out]
        n152 = disable-structure shown="Disabled" {
          frame Disabled {
            n153 = local read "Path"() -> (w183:path)
            n154 = control-ref of="PT mag"() -> (w182:refnum<vi>)
            n155 = control-ref of="PT phase"() -> (w181:refnum<vi>)
            n156 = call "Calibration Smoothing Tool.vi"("Path In"=w183) -> ("Smoothed?"=w184:bool)  [unwired: 10 in]
            n157 = case shown="True" w184 {
              tunnel: w183 -> [_ w187]
              tunnel: w182 -> [_ w189]
              tunnel: w181 -> [_ w188]
              frame False {
              }
              frame True {
                w191 = cluster{"PTC Mag":dbl[], "PTC Phase":dbl[]}[] [] ("PT mag graph")
                n158 = property on="Property Node" class="XYGraph (strict)"(reference=w188, "Value"=w191) -> (reference out=w185:refnum<vi>)  [unwired: 1 in, 1 out]
                n159 = property on="Property Node" class="XYGraph (strict)"(reference=w189, "Value"=w191, "Legend Visible"=FALSE ("Legend:Visible")) -> (reference out=w186:refnum<vi>)  [unwired: 1 in, 1 out]
                n160 = call "CAL-Plot Data.vi"("Path"=w187, "Name"=w186, 7:w185) -> ()  [unwired: 11 in, 2 out]
              }
            }
          }
          frame Enabled {
          }
        }
      }
      event "Validate Button": Value Change {
        n161 = event-data() -> ()  [unwired: 1 in, 1 out]
        n162 = disable-structure shown="Disabled" {
          frame Disabled {
            n163 = local read "Probe Mic Gain (dB)"() -> (w196:dbl)
            n164 = local read "Cal Mic Sens"() -> (w194:dbl)
            n165 = local read "Cal Mic Gain (dB)"() -> (w195:dbl)
            n166 = local read "Path"() -> (w199:path)
            n167 = local read "Ear"() -> (w193:enum16{"Right", "Left"})
            n168 = call "FileIO-File or Folder Exists.vi"("path"=w199) -> ("Exists?"=w198:bool, "dup path"=w197:path)  [unwired: 7 in, 2 out]
            n169 = case shown="True" w198 {
              tunnel: w197 -> [_ w204]
              tunnel: w196 -> [_ w203]
              tunnel: w195 -> [_ w202]
              tunnel: w194 -> [_ w201]
              tunnel: w193 -> [_ w200]
              frame False {
              }
              frame True {
                n170 = call "Cal Validation.vi"("Path In"=w204, "Probe Mic Gain (dB)"=w203, "Cal Mic Gain (dB)"=w202, "Cal Mic Sens (dB)"=w201, "Ear"=w200) -> ()  [unwired: 11 in]
              }
            }
          }
          frame Enabled {
          }
        }
      }
    }
  }
